vi "Get Image Portion.vi"(5 "h":i16, 7 "w":i16, 8 "error in (no error)":errorcluster, 9 "y":i16, 10 "x":i16, 11 "path":path) -> (0 "error out":errorcluster)   [LabVIEW 2023]
uses:
  System.Drawing
  labview_win_util32_8.6/WINUTIL.LLB/Extract Window Origin / Size.vi
panel:
  in  "window name":string
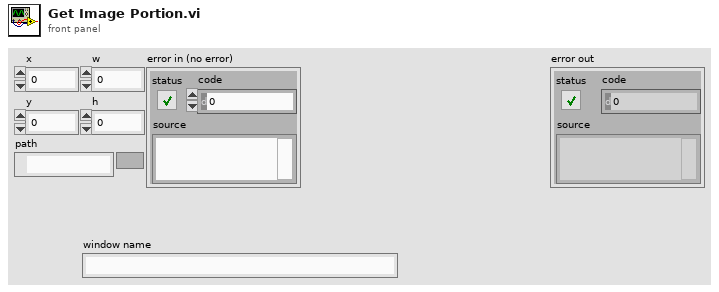
[diagram p1: front panel]
types:
  T1 = typedef "Window Refnum" = refnum<k1>
  T2 = typedef "Window Rectangle.ctl" = cluster{"left":i16, "top":i16, "right":i16, "bottom":i16}
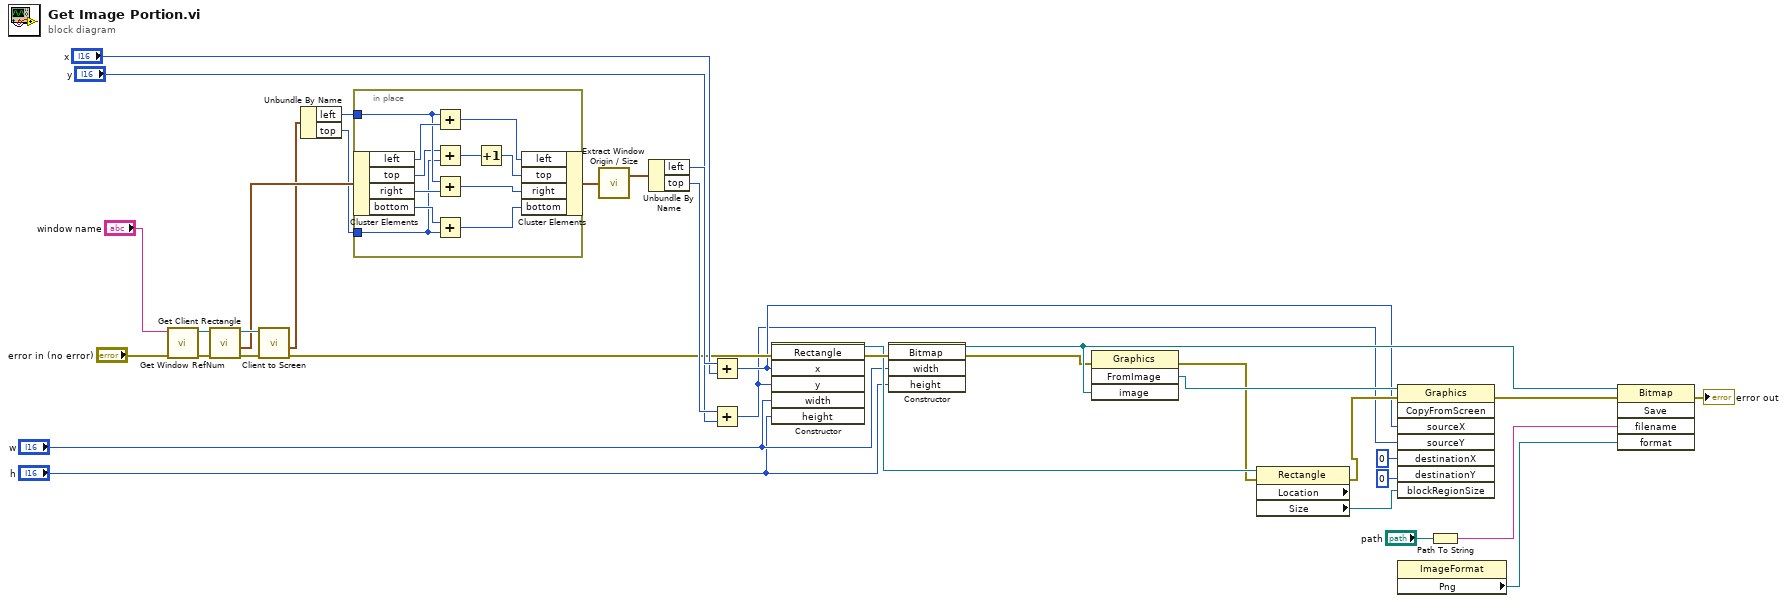
[diagram p0: block diagram]
diagram:
  n1 = call "Get Window RefNum.vi"("error in (no error)"="error in (no error)", "window name (\"\")"="window name") -> ("error out"=w36:errorcluster, "window refnum (NaWR)"=w35:T1)  [unwired: 6 in]
  n2 = call "Get Client Rectangle.vi"("error in (no error)"=w36, "window refnum (NaWR)"=w35) -> ("error out"=w27:errorcluster, "window rect"=w25:T2, "window refnum out"=w26:T1)  [unwired: 3 in]
  n3 = call "Client to Screen.vi"("error in (no error)"=w27, "window refnum (NaWR)"=w26) -> ("error out"=w10:errorcluster, "window point"=w24:cluster{"left":i16, "top":i16})  [unwired: 3 in, 1 out]
  n4 = Unbundle By Name(w24) -> ("left"=w23:i16, "top"=w21:i16)
  n5 = in-place {
    in-place-border: w23 -> [w45]
    in-place-border: w21 -> [w42]
    n6 = in-place-cluster #1(w25) -> ("left"=w47:i16, "top"=w44:i16, "right"=w46:i16, "bottom"=w43:i16)
    n7 = Add(x=w45, y=w47) -> (x+y=w41:i16)
    n8 = Add(x=w44, y=w42) -> (x+y=w40:i16)
    n9 = Add(x=w45, y=w46) -> (x+y=w39:i16)
    n10 = Add(x=w43, y=w42) -> (x+y=w38:i16)
    n11 = Increment(x=w40) -> (x+1=w37:i16)
    n12 = in-place-cluster #1("left"=w41, "top"=w37, "right"=w39, "bottom"=w38) -> (w22:T2)
  }
  n13 = call "Extract Window Origin / Size.vi"("window rect"=w22) -> ("window origin"=w28:cluster{"left":i16, "top":i16})  [unwired: 1 out]
  n14 = Unbundle By Name(w28) -> ("left"=w32:i16, "top"=w31:i16)
  n15 = Add(x=w32, y="x") -> (x+y=w6:i16)
  n16 = Add(x=w31, y="y") -> (x+y=w5:i16)
  n17 = constructor class="Rectangle"(error in=w10, "x"=w6, "y"=w5, "width"="w", "height"="h") -> (reference out=w33:refnum<k24>, error out=w34:errorcluster)  [unwired: 2 in, 5 out]
  n18 = constructor class="Bitmap"(error in=w34, "width"="w", "height"="h") -> (reference out=w29:refnum<k24>, error out=w9:errorcluster)  [unwired: 2 in, 3 out]
  n19 = invoke class="Graphics" method="FromImage"(error in=w9, "image"=w29) -> (error out=w8:errorcluster, "FromImage"=w13:refnum<k24>)  [unwired: 2 in, 2 out]
  n20 = property class="Rectangle" props=["Location", "Size"](reference=w33, error in=w8) -> (error out=w7:errorcluster, "Size"=w2:refnum<k24>)  [unwired: 2 out]
  n21 = invoke class="Graphics" method="CopyFromScreen"(reference=w13, error in=w7, "sourceX"=w6, "sourceY"=w5, "destinationX"=0, "destinationY"=0, "blockRegionSize"=w2) -> (error out=w15:errorcluster)  [unwired: 1 in, 7 out]
  n22 = property class="ImageFormat"() -> ("Png"=w16:refnum<k24>)  [unwired: 2 in, 2 out]
  n23 = Path To String(path="path") -> (string=w30:string)
  n24 = invoke class="Bitmap" method="Save"(reference=w29, error in=w15, "filename"=w30, "format"=w16) -> (error out=→"error out":errorcluster)  [unwired: 1 in, 4 out]
